vi "Get Test Group.vi"(8 "error in (no error)":errorcluster, 10 "Test Group Name":string, 11 "Test Group Manager in":refnum<class "Test Group Manager.lvclass">) -> (0 "error out":errorcluster, 2 "Test Group In":refnum<data-value>, 3 "Test Group Manager out":refnum<class "Test Group Manager.lvclass">)   [LabVIEW 2016, in "Test Group Manager.lvlib" / "Test Group Manager.lvclass"]
uses:
  Test Group Manager.lvclass
  Includes/Test Group/Test Group.lvclass
  Test Group Manager.lvclass/Test Group Manager.ctl
  Protected Methods/Read Test Group Database.vi
  <vilib>/Utility/error.llb/Error Cluster From Error Code.vi
  <vilib>/ErrorRing/Error Ring.xnode
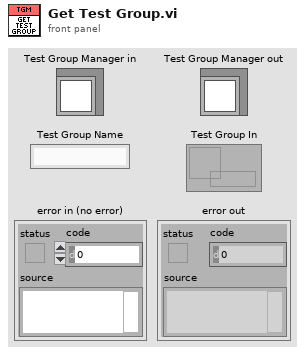
[diagram p1: front panel]
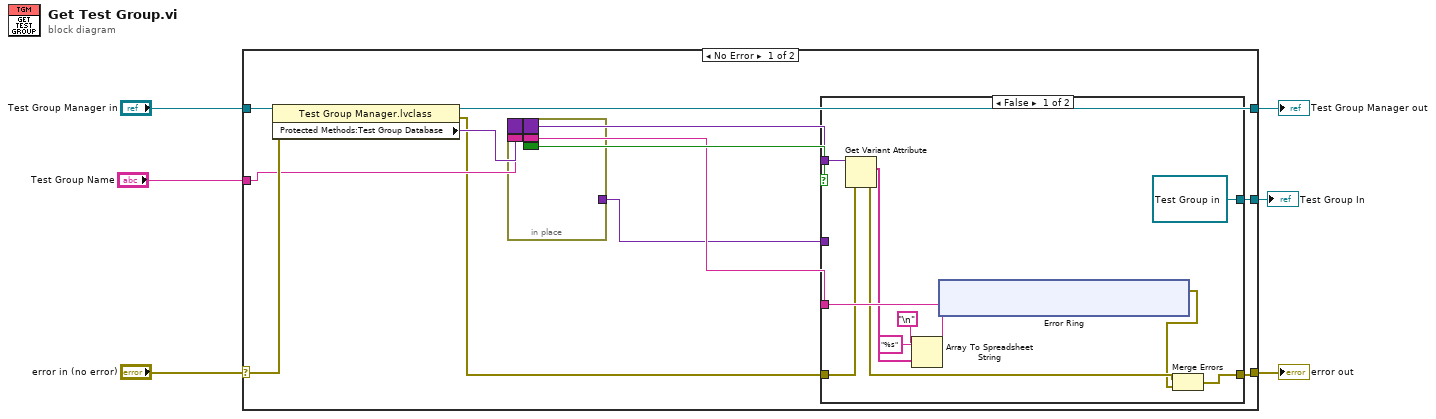
[diagram p0: block diagram]
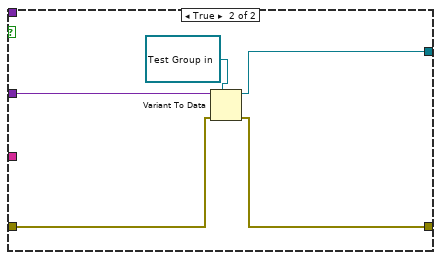
[diagram p2: hidden frame]
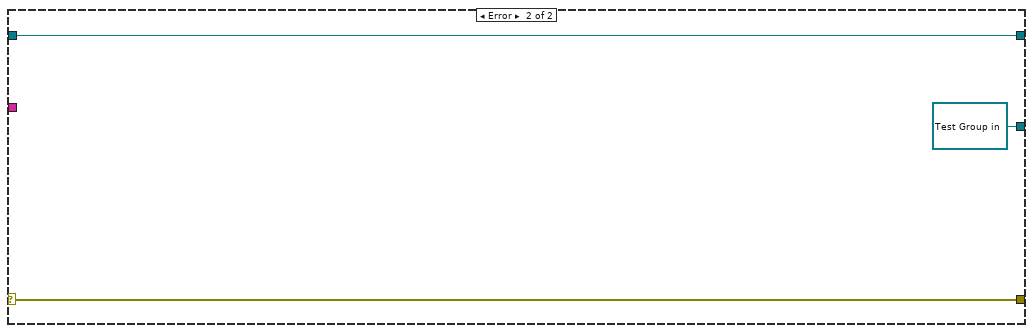
[diagram p3: hidden frame]
diagram:
  n1 = case shown="No Error" "error in (no error)" {
    selector: "error in (no error)" -> [w18 w46]
    tunnel: [w12 w46] -> w5
    tunnel: [w16 w45] -> w3
    tunnel: "Test Group Manager in" -> [w17 w45]
    tunnel: "Test Group Name" -> [w14 _]
    tunnel: [w7 refnum<data-value> refnum ("Test Group In")] -> w1
    frame No Error {
      n2 = property class="Test Group Manager.lvclass"(reference=w17, error in=w18) -> (reference out=w16:refnum<class "Test Group Manager.lvclass">, error out=w8:errorcluster, "Protected Methods:Test Group Database"=w15:variant)
      n3 = in-place {
        border: w15 -> [_]
        border: w14 -> [_]
        border: [_] -> w10
        border: [_] -> w11
        border: [_] -> w13
        in-place-border: [w43] -> w9
      }
      n4 = case shown="False" w13 {
        tunnel: [w28 w39] -> w12
        tunnel: w8 -> [w26 w40]
        tunnel: w11 -> [w29 _]
        tunnel: w10 -> [w27 _]
        tunnel: w9 -> [_ w41]
        tunnel: [refnum<data-value> refnum ("data value reference") w38] -> w7
        frame False {
          n5 = Get Variant Attribute(Variant=w27, error in=w26) -> (names=w24:string[], error out=w25:errorcluster)  [unwired: 2 in, 2 out]
          n6 = Array To Spreadsheet String(delimiter (Tab)="\n", array=w24, 3:"%s" ("format string")) -> (spreadsheet string=w21:string)
          n7 = xnode "Error Ring"("parameter 0"=w29, "parameter 1"=w21) -> ("error out"=w20:errorcluster)
          n8 = Merge Errors(w25, w20) -> (w28:errorcluster)
        }
        frame True {
          n9 = Variant To Data(error in=w40, type=refnum<data-value> refnum ("data value reference"), Variant=w41) -> (data=w38:refnum<data-value>, error out=w39:errorcluster)
        }
      }
    }
    frame Error {
    }
  }
  "error out" <- w5
  "Test Group Manager out" <- w3
  "Test Group In" <- w1
